vi "labview_results_get.vi"(0 "Path":path, 1 "Dust ID":string, 5 "Upper Timestamp":dbl, 7 "Velocity Limits":cluster{dbl, dbl}, 8 "Lower Timestamp":dbl, 12 "Particle Quality":cluster{i32, i32}, 14 "Session Quality":cluster{i32, i32}, 15 "Experiment ID":string, 17 "Dust Material":string) -> (20 "Results Output":string, 21 "Results Error/Debug":string, 25 "Request":string)   [LabVIEW 2015]
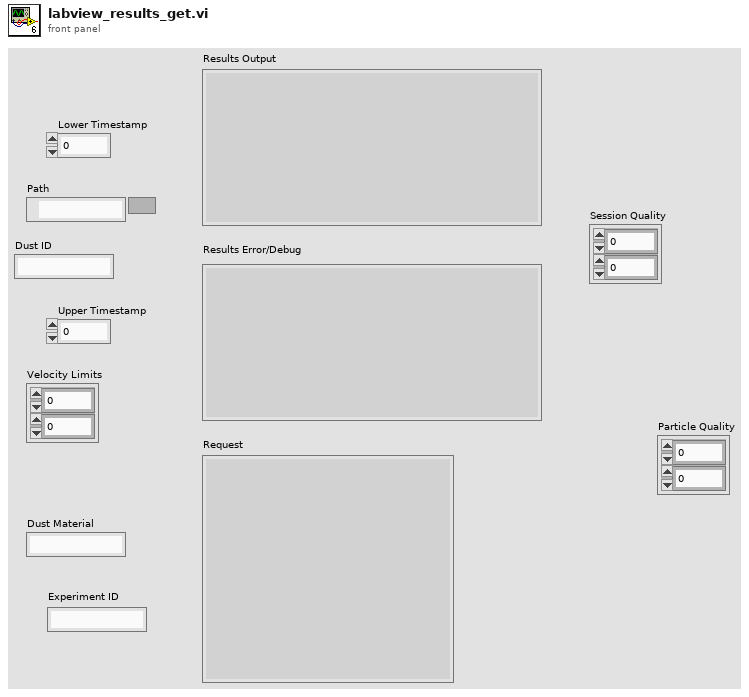
[diagram p1: front panel]
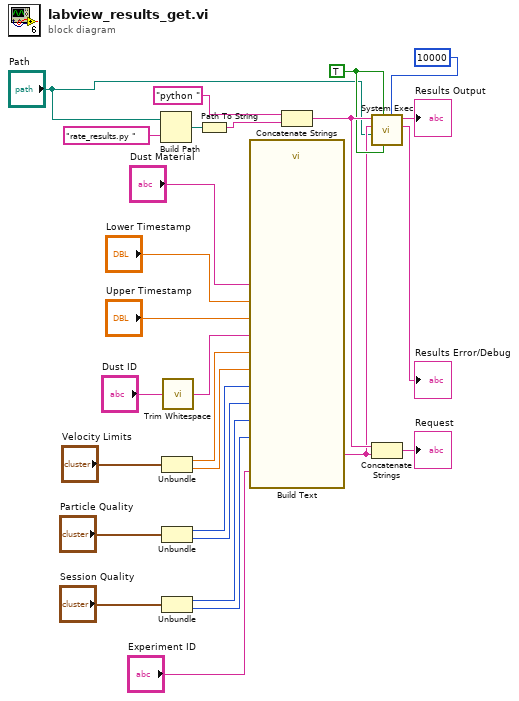
[diagram p0: block diagram]
diagram:
  w22 = TRUE
  n1 = Build Path(base path="Path", name or relative path="rate_results.py ") -> (appended path=w4:path)
  n2 = Unbundle("Velocity Limits") -> (w16:dbl, w15:dbl)
  n3 = Unbundle("Particle Quality") -> (w10:i32, w9:i32)
  n4 = Unbundle("Session Quality") -> (w13:i32, w12:i32)
  n5 = call <vilib>:"Trim Whitespace.vi"("string"="Dust ID") -> ("trimmed string"=w18:string)  [unwired: 1 in]
  n6 = Path To String(path=w4) -> (string=w3:string)
  n7 = call "Build Text"("start"="Lower Timestamp", "stop"="Upper Timestamp", "dustID"=w18, "vmin"=w16, "vmax"=w15, "material"="Dust Material", "pq_min"=w10, "pq_max"=w9, "sq_min"=w13, "sq_max"=w12, "experiment_ID"="Experiment ID") -> ("Result"=w17:string)  [unwired: 15 in, 1 out]
  n8 = Concatenate Strings("python ", w3) -> (w26:string)
  n9 = call <vilib>:"System Exec.vi"("expected output size  (4096)"=10000, "run minimized? (F)"=w22, "wait until completion? (T)"=w22, "working directory"="Path", "standard input"=w17, "command line"=w26) -> ("standard error"=→"Results Error/Debug":string, "standard output"=→"Results Output":string)  [unwired: 2 in, 2 out]
  n10 = Concatenate Strings(w26, w17) -> (→"Request":string)
